vi "Generator ZKP.vi"(8 "error in":errorcluster) -> (0 "error out":errorcluster)   [LabVIEW 2014]
doc: "This VI generates a given acoustic signal using the sound card.\n\n---------------------\npawlik@agh.edu.pl\n01.04.2019"
uses:
  Generator ZKP/states.ctl
  <vilib>/sound2/lvsound2.llb/Sound Data Format.ctl
  <vilib>/sound2/lvsound2.llb/Sound Output Task ID.ctl
  <vilib>/sound2/lvsound2.llb/Sound Output Write (DBL Single).vi
  <vilib>/addons/_NISVFA/_Generation/SoundVib_Generation.lvlib
  <vilib>/measure/NI_MABase.lvlib
panel:
  out "signal":waveform(dbl)(graph)
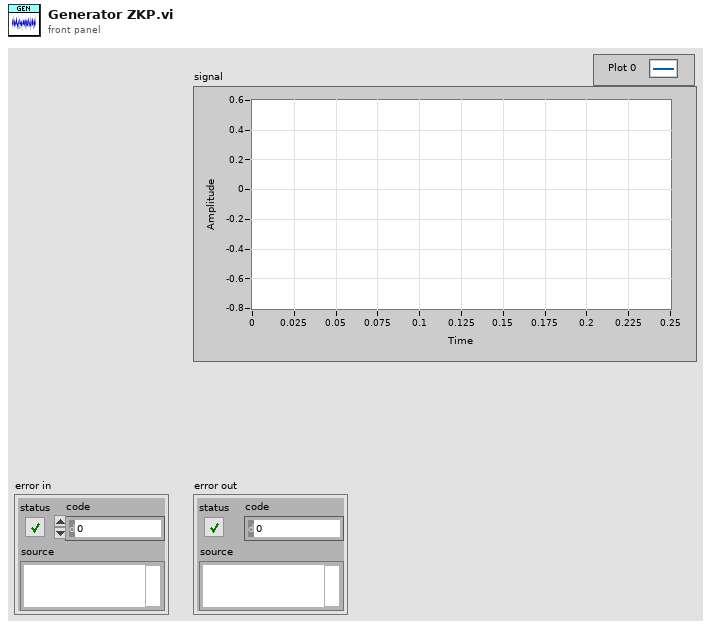
[diagram p1: front panel]
types:
  T1 = typedef "Sound Data Format.ctl" = cluster{"sample rate (S/s)":dbl, "number of channels":i32, "bits per sample":i32}
  T2 = typedef "states.ctl" = enum16{"Idle", "Init", "Generate", "Stop", "Exit"}
  T3 = typedef "Sound Output Task ID.ctl" = u32
  T4 = typedef "Generator_ZKP_Parametry.ctl" = cluster{"Parametry sygnału":T5, "Rodzaj sygnału":T6, "command":T7}
  T5 = typedef "signal parameters.ctl" = cluster{"amplitude":dbl, "chirp duration [s]":dbl, "frequency range":cluster{"start frequency [Hz]":dbl, "stop frequency [Hz]":dbl}}
  T6 = typedef "signal type.ctl" = enum16{"pink noise", "white noise", "chirp"}
  T7 = typedef "command.ctl" = enum16{"play", "stop", "exit"}
  T8 = cluster{"start frequency [Hz]":dbl, "stop frequency [Hz]":dbl}
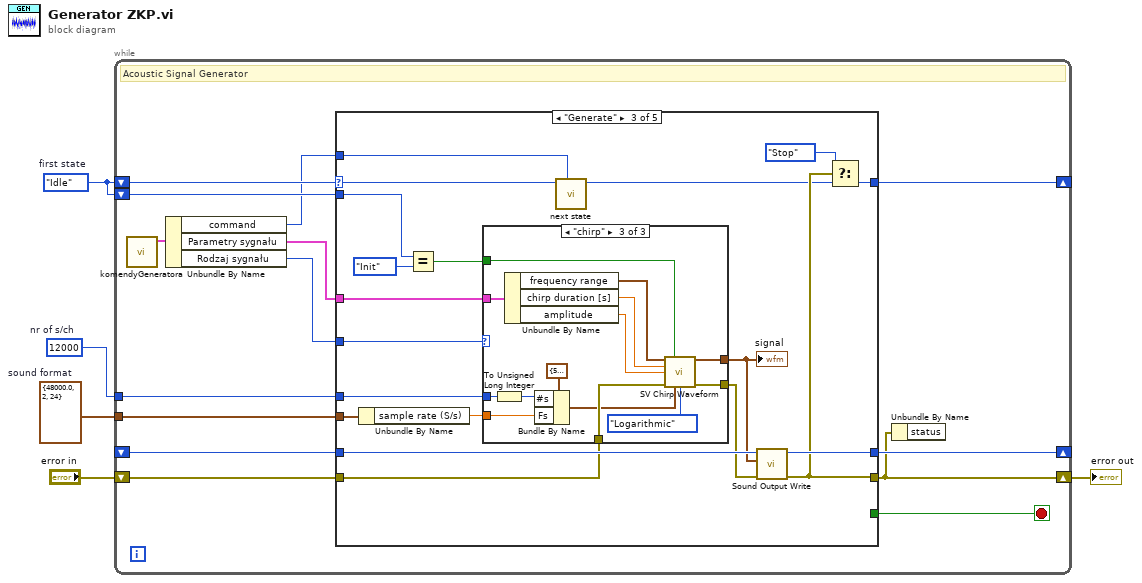
[diagram p0: block diagram]
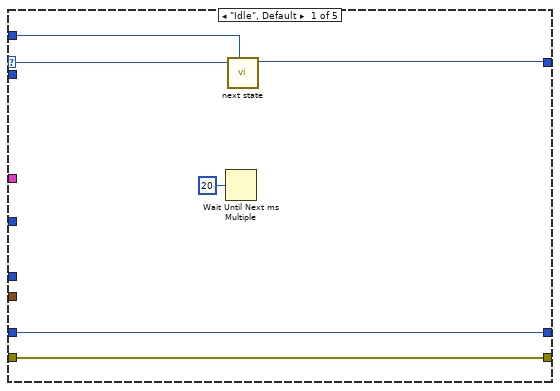
[diagram p2: hidden frame]
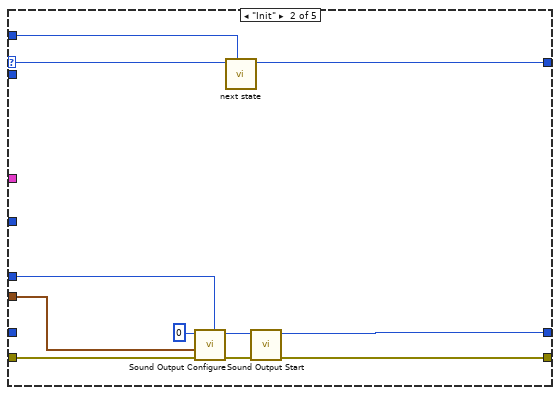
[diagram p3: hidden frame]
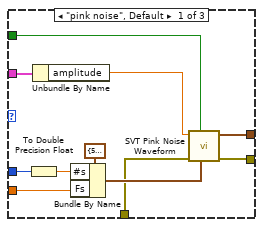
[diagram p4: hidden frame]
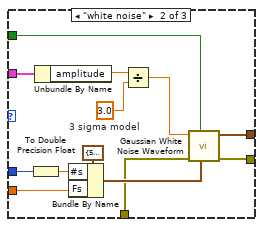
[diagram p5: hidden frame]
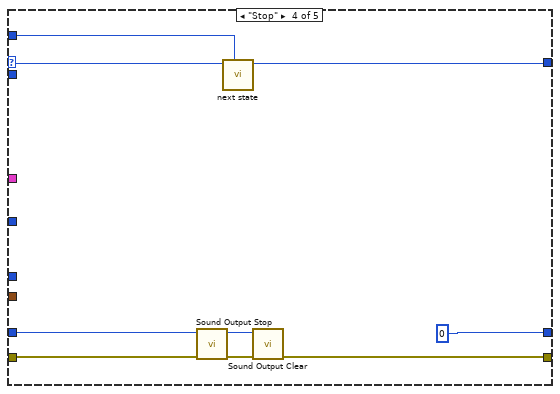
[diagram p6: hidden frame]
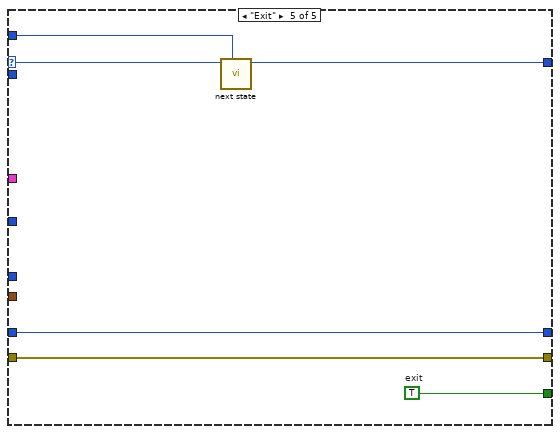
[diagram p7: hidden frame]
diagram:
  w4 = T1 {"sample rate (S/s)"=48000.0, "number of channels"=2, "bits per sample"=24}  # sound format
  w5 = 12000  # nr of s/ch
  w3 = states."Idle"  # first state
  n1 = while {
    shift-right: [w18] -> _
    shift-left: w3 -> [w19]
    shift-right: [w17] -> _
    shift-left: _ -> [w15]
    shift-right: [w7] -> w2
    shift-left: "error in" -> [w16]
    tunnel: w5 -> [w14]
    tunnel: w4 -> [w13]
    shift-left: w3 -> [w12]
    stop <- w8 stop-if-true
    # "Acoustic Signal Generator"
    n2 = call "komendyGeneratora.vi"() -> ("Generator_ZKP_Wyjście"=w6:T4)  [unwired: 11 in]
    n3 = Unbundle By Name(w6) -> ("command"=w11:T7, "Parametry sygnału"=w10:T5, "Rodzaj sygnału"=w9:T6)
    n4 = case shown="\"Generate\"" w19 {
      selector: w19 -> [w22 w28 w42 w95 w108]
      tunnel: [w21 w27 w38 w96 w107] -> w18
      tunnel: [w25 w33 w55 T3 0 ("task ID out") w104] -> w17
      tunnel: [w24 w32 w40 w98 w105] -> w7
      tunnel: w16 -> [w24 w30 w44 w100 w105]
      tunnel: w14 -> [_ w31 w43 _ _]
      tunnel: w15 -> [w25 _ w54 w101 w104]
      tunnel: w13 -> [_ w29 w53 _ _]
      tunnel: w9 -> [_ _ w52 _ _]
      tunnel: w12 -> [_ _ w50 _ _]
      tunnel: w10 -> [_ _ w46 _ _]
      tunnel: w11 -> [w20 w26 w41 w94 w106]
      tunnel: [_ _ _ _ w103] -> w8
      frame "Idle", Default {
        n5 = Wait Until Next ms Multiple(millisecond multiple=u32 20 ("milliseconds to wait")) -> ()  [unwired: 1 out]
        n6 = call "next state.vi"("command"=w20, "actual state"=w22) -> ("next state"=w21:T2)  [unwired: 9 in]
      }
      frame "Init" {
        n7 = call <vilib>:"Sound Output Configure.vi"("number of samples/ch"=w31, "error in (no error)"=w30, "sound format"=w29, "device ID"=u32 0) -> ("error out"=w35:errorcluster, "task ID"=w36:T3)  [unwired: 6 in]
        n8 = call "next state.vi"("command"=w26, "actual state"=w28) -> ("next state"=w27:T2)  [unwired: 9 in]
        n9 = call <vilib>:"Sound Output Start.vi"("error in (no error)"=w35, "task ID"=w36) -> ("error out"=w32:errorcluster, "task ID out"=w33:T3)  [unwired: 8 in]
      }
      frame "Generate" {
        n10 = Unbundle By Name(w53) -> ("sample rate (S/s)"=w47:dbl)
        n11 = Equal?(x=w50, y=states."Init") -> (x = y?=w48:bool)
        n12 = case shown="\"chirp\"" w52 {
          tunnel: [w66 w79 w93] -> w51
          tunnel: w48 -> [w65 w78 w91]
          tunnel: w47 -> [w63 w76 w84]
          tunnel: w46 -> [w61 w74 w90]
          tunnel: [w58 w70 w86] -> w45
          tunnel: w44 -> [w59 w69 w85]
          tunnel: w43 -> [w57 w68 w83]
          frame "pink noise", Default {
            n13 = To Double Precision Float(number=w57) -> (double precision float=w56:dbl)
            n14 = Unbundle By Name(w61) -> ("amplitude"=w60:dbl)
            n15 = Bundle By Name(cluster=cluster{"Fs":dbl, "#s":dbl} {"Fs"=51200.0, "#s"=1024.0} ("sampling info"), "#s"=w56, "Fs"=w63) -> (w62:cluster{"Fs":dbl, "#s":dbl})
            n16 = call <vilib>:"SVT Pink Noise Waveform.vi"("sampling info"=w62, "reset signal (F)"=w65, "error in (no error)"=w59, "amplitude"=w60) -> ("error out"=w58:errorcluster, "pink noise signal"=w66:waveform(dbl))  [unwired: 6 in]
          }
          frame "white noise" {
            w72 = 3.0  # 3 sigma model
            n17 = To Double Precision Float(number=w68) -> (double precision float=w67:dbl)
            n18 = Unbundle By Name(w74) -> ("amplitude"=w73:dbl)
            n19 = Bundle By Name(cluster=cluster{"Fs":dbl, "#s":dbl} {"Fs"=51200.0, "#s"=1024.0} ("sampling info"), "#s"=w67, "Fs"=w76) -> (w75:cluster{"Fs":dbl, "#s":dbl})
            n20 = Divide(x=w73, y=w72) -> (x/y=w71:dbl)
            n21 = call <vilib>:"Gaussian White Noise Waveform.vi"("sampling info"=w75, "reset signal"=w78, "error in (no error)"=w69, "standard deviation"=w71) -> ("error out"=w70:errorcluster, "signal out"=w79:waveform(dbl))  [unwired: 6 in]
          }
          frame "chirp" {
            n22 = To Unsigned Long Integer(number=w83) -> (unsigned 32bit integer=w80:u32)
            n23 = Unbundle By Name(w90) -> ("frequency range"=w89:T8, "chirp duration [s]"=w88:dbl, "amplitude"=w87:dbl)
            n24 = Bundle By Name(cluster=cluster{"Fs":dbl, "#s":u32} {"Fs"=51200.0, "#s"=1024} ("sampling info"), "#s"=w80, "Fs"=w84) -> (w81:cluster{"Fs":dbl, "#s":u32})
            n25 = call <vilib>:"SV Chirp Waveform.vi"("frequency range"=w89, "reset signal (F)"=w91, "chirp duration [s]"=w88, "amplitude"=w87, "error in (no error)"=w85, "sampling info"=w81, "frequency spacing"=enum16{"Linear", "Logarithmic"}."Logarithmic") -> ("chirp signal"=w93:waveform(dbl), "error out"=w86:errorcluster)  [unwired: 6 in, 1 out]
          }
        }
        "signal" <- w51
        n26 = call "next state.vi"("command"=w41, "actual state"=w42) -> ("next state"=w39:T2)  [unwired: 9 in]
        n27 = call-poly <vilib>:"Sound Output Write.vi"("error in (no error)"=w45, "data"=w51, "task ID"=w54) -> ("error out"=w40:errorcluster, "task ID out"=w55:T3)  [unwired: 7 in]
        n28 = Select(t=states."Stop", s=w40, f=w39) -> (s? t:f=w38:T2)
      }
      frame "Stop" {
        n29 = call <vilib>:"Sound Output Stop.vi"("error in (no error)"=w100, "task ID"=w101) -> ("error out"=w102:errorcluster, "task ID out"=w99:T3)  [unwired: 8 in]
        n30 = call "next state.vi"("command"=w94, "actual state"=w95) -> ("next state"=w96:T2)  [unwired: 9 in]
        n31 = call <vilib>:"Sound Output Clear.vi"("error in (no error)"=w102, "task ID"=w99) -> ("error out"=w98:errorcluster)  [unwired: 9 in]
      }
      frame "Exit" {
        w103 = TRUE  # exit
        n32 = call "next state.vi"("command"=w106, "actual state"=w108) -> ("next state"=w107:T2)  [unwired: 9 in]
      }
    }
    n33 = Unbundle By Name(w7) -> ()  [unwired: 1 out]
  }
  "error out" <- w2
